vi "Read refnum.vi"(8 "error in (no error)":errorcluster, 11 "DataWriter in":refnum<class "DataWriter.lvclass">) -> (0 "error out":errorcluster, 2 "refnum":refnum<file>, 3 "DataWriter out":refnum<class "DataWriter.lvclass">)   [LabVIEW 2024, in "Data.lvlib" / "DataWriter.lvclass"]
uses:
  DataWriter.lvclass
  DataWriter.lvclass/DataWriter.ctl
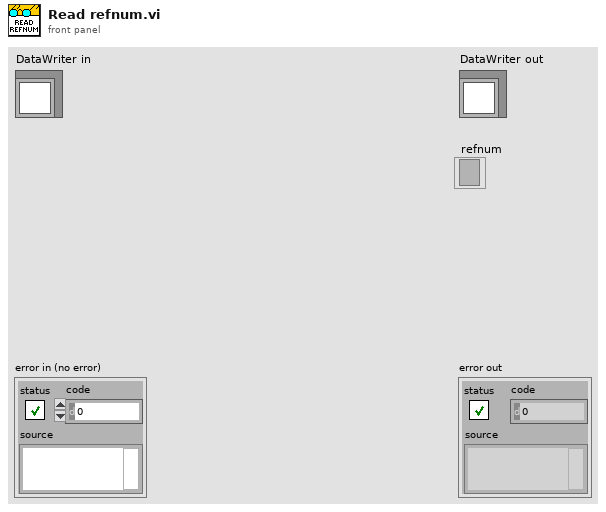
[diagram p1: front panel]
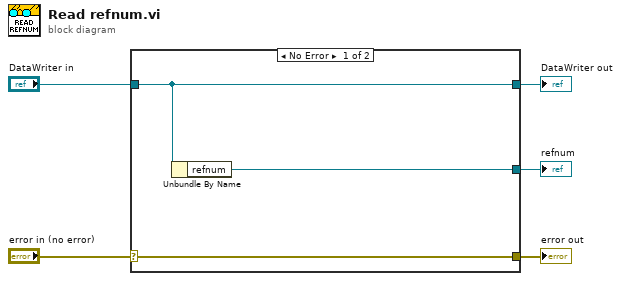
[diagram p0: block diagram]
diagram:
  n1 = case shown="No Error" "error in (no error)" {
    selector: "error in (no error)" -> [w8 w9]
    tunnel: [w8 w9] -> w4
    tunnel: [w7 w10] -> w2
    tunnel: "DataWriter in" -> [w7 w10]
    tunnel: [w6 _] -> w1
    frame No Error {
      n2 = Unbundle By Name(w7) -> ("refnum"=w6:refnum<file>)
    }
    frame Error {
    }
  }
  "error out" <- w4
  "DataWriter out" <- w2
  "refnum" <- w1
